vi "P4CMDSub Get Env Info.vi"() -> (1 "user":string, 2 "client":string, 3 "port":string, 5 "command output":string)   [LabVIEW 2017, in "NI_SCC_P4CMD.lvlib"]
uses:
  <vilib>/SourceControl/Providers/P4CMD/NI_SCC_P4CMD.lvlib
  <vilib>/SourceControl/Providers/P4CMD/P4CMD Operations.ctl
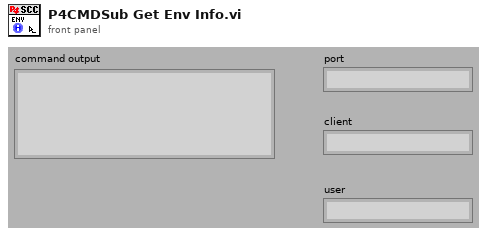
[diagram p1: front panel]
types:
  T1 = typedef "NI_SCC_P4CMD.lvlib/P4CMD Operations.ctl" = enum16{"get all clients", "get all users", "describe changelist", "sync from depot", "open for edit", "submit to depot", "revert", "add to depot", "remove from depot", "print files revisions", "compare client file", "print depot file contents", "list opened files", "get file info", "lock files", "edit changelist spec", "info", "set variables"}
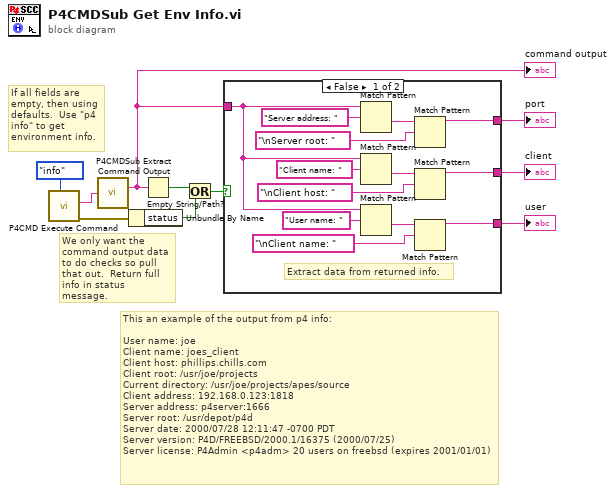
[diagram p0: block diagram]
diagram:
  # "We only want the command output data to do checks so pull that out.  Return full info in status message."
  # "This an example of the output from p4 info:\n\nUser name: joe\nClient name: joes_client\nClient host: phillips.chills.com\nClient root: /usr/joe/projects\nCurrent directory: /usr/joe/projects/apes/source\nClient address: 192.168.0.123:1818\nServer address: p4server:1666\nServer root: /usr/depot/p4d\nServer date: 2000/07/28 12:11:47 -0700 PDT\nServer version: P4D/FREEBSD/2000.1/16375 (2000/07/25)\nServer license: P4Admin <p4adm> 20 users on freebsd (expires 2001/01/01)"
  # "If all fields are empty, then using defaults.  Use \"p4 info\" to get environment info."
  n1 = call <vilib>:"P4CMD Execute Command.vi"("p4 operation"=P4CMD_Operations."info") -> ("error out"=w8:errorcluster, "command information"=w9:string)  [unwired: 8 in, 1 out]
  n2 = call <vilib>:"P4CMDSub Extract Command Output.vi"("bundled message"=w9) -> ("command output"=w10:string)  [unwired: 13 in, 1 out]
  "command output" <- w10
  n3 = Unbundle By Name(w8) -> ("status"=w1:bool)
  n4 = Empty String/Path?(string/path=w10) -> (empty?=w2:bool)
  n5 = Or(x=w2, y=w1) -> (x .or. y?=w3:bool)
  n6 = case shown="False" w3 {
    tunnel: w10 -> [w12 _]
    tunnel: [w20 _] -> w4
    tunnel: [w16 _] -> w5
    tunnel: [w11 _] -> w6
    frame False {
      # "Extract data from returned info."
      n7 = Match Pattern(string=w12, regular expression="Server address: " ("command line")) -> (after substring=w22:string)  [unwired: 1 in, 3 out]
      n8 = Match Pattern(string=w12, regular expression="Client name: " ("command line")) -> (after substring=w17:string)  [unwired: 1 in, 3 out]
      n9 = Match Pattern(string=w12, regular expression="User name: " ("command line")) -> (after substring=w15:string)  [unwired: 1 in, 3 out]
      n10 = Match Pattern(string=w22, regular expression="\nServer root: " ("command line")) -> (before substring=w20:string)  [unwired: 1 in, 3 out]
      n11 = Match Pattern(string=w17, regular expression="\nClient host: " ("command line")) -> (before substring=w16:string)  [unwired: 1 in, 3 out]
      n12 = Match Pattern(string=w15, regular expression="\nClient name: " ("command line")) -> (before substring=w11:string)  [unwired: 1 in, 3 out]
    }
    frame True {
    }
  }
  "user" <- w6
  "client" <- w5
  "port" <- w4
